vi "TC_signal.vi"() -> ()   [LabVIEW 2018]
uses:
  tc_type.ctl
panel:
  out "Graphe XY":T1(graph)
  in  "Thermocouple":T2=5 items=["B", "E", "J", "K", "R", "S", "T", "N"]
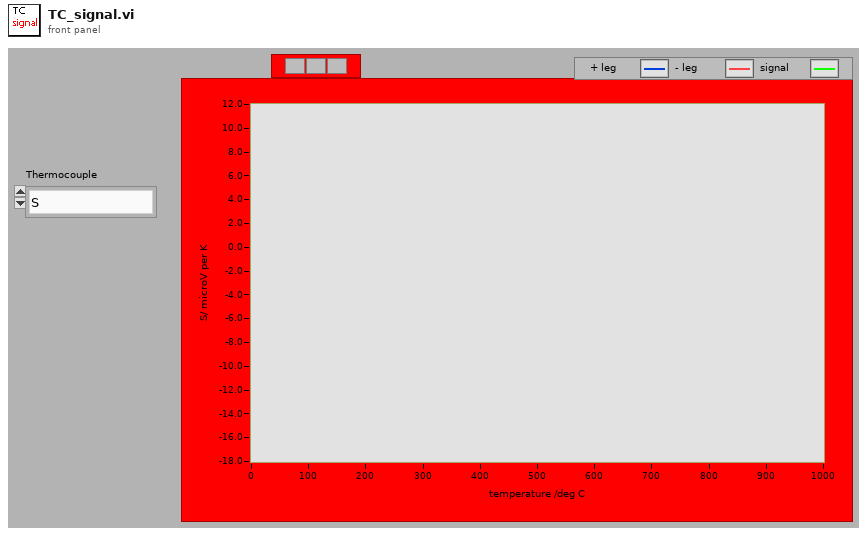
[diagram p1: front panel]
types:
  T1 = cluster{cluster{i32, "S of - wire /microV/K":dbl}[]}[]
  T2 = typedef "tc_type.ctl" = u16
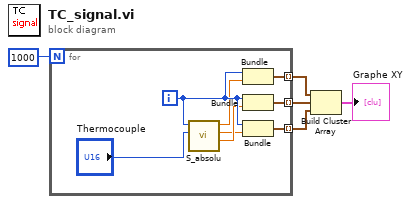
[diagram p0: block diagram]
diagram:
  n1 = for {
    N: 1000 -> [_]
    tunnel: [w12] -> w4 mode=indexing
    tunnel: [w8] -> w2 mode=indexing
    tunnel: [w7] -> w1 mode=indexing
    i -> [w13]
    n2 = call "S_absolu.vi"("Th  (Seebeck)"="Thermocouple", "T, in  Kelvin"=w13) -> ("TC signal /microVperK"=w10:dbl, "S of - wire /microV/K"=w9:dbl, "S of + wire /microV/K"=w11:dbl)  [unwired: 7 in]
    n3 = Bundle(w13, "S of + wire /microV/K"=w11) -> (w12:cluster{i32, "S of + wire /microV/K":dbl})  [unwired: 1 out]
    n4 = Bundle(w13, "TC signal /microVperK"=w10) -> (w8:cluster{i32, "TC signal /microVperK":dbl})  [unwired: 1 out]
    n5 = Bundle(w13, "S of - wire /microV/K"=w9) -> (w7:cluster{i32, "S of - wire /microV/K":dbl})  [unwired: 1 out]
  }
  n6 = Build Cluster Array(w4, w2, w1) -> (→"Graphe XY":T1)
